vi "test Failing.vi"(8 "error in (no error)":errorcluster, 11 "Dummy In":refnum<class "Dummy.lvclass">) -> (0 "error out":errorcluster, 3 "Dummy Out":refnum<class "Dummy.lvclass">)   [LabVIEW 2020, in "Dummy.lvclass"]
doc: "Failing test"
uses:
  Dummy.lvclass
  C:/git/astemes-lunit/source/Framework/Test Case/LUnit Test Case.lvclass
  Framework/Test Case/LUnit Test Case.lvclass/LUnit Test Case.ctl
  Framework/Test Case/Private/SubVIs/Set Assertion Type.vi
  Framework/Test Case/Assertions/Pass.vi
  Framework/Test Case/Assertions/Fail.vi
  Framework/Test Case/Private/SubVIs/Add test result.vi
  Framework/Result Types/Case Result/Public/Record Assertion Result.vi
  Framework/Result Types/Method Result/Public/Aggregate Assertion Results.vi
  Framework/Result Types/Method Result/Private/Merge Status.vi
  Framework/Result Types/Method Result/Private/Concatenate result strings.vi
  Framework/Test Case/LUnit Test Case.lvclass
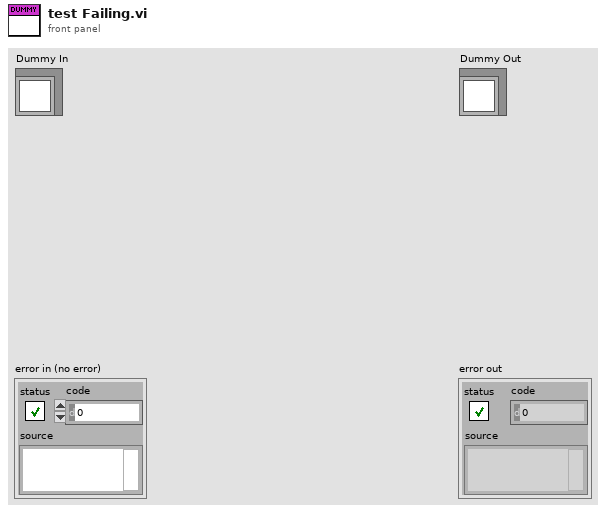
[diagram p1: front panel]
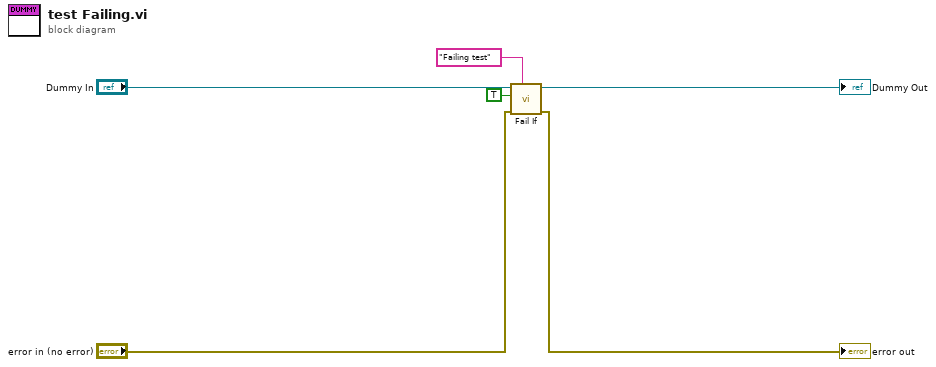
[diagram p0: block diagram]
diagram:
  n1 = call "Fail If.vi"("Description"="Failing test", "error in (no error)"="error in (no error)", "Fail?"=TRUE ("Pass?"), "LUnit Test Case In"="Dummy In") -> ("error out"=→"error out":errorcluster, "LUnit Test Case Out"=→"Dummy Out":refnum<class "Dummy.lvclass">)  [unwired: 6 in]
